vi "tm_setparameterByName.vi"(8 "error in (no error)":errorcluster, 9 "Value":dbl, 10 "Parameter Name":string, 11 "Handle in":u32) -> (0 "error out":errorcluster, 1 "Value out":dbl, 3 "Handle out":u32)   [LabVIEW 2021, in "Camera.lvlib" / "Camera.lvclass"]
uses:
  Camera.lvclass
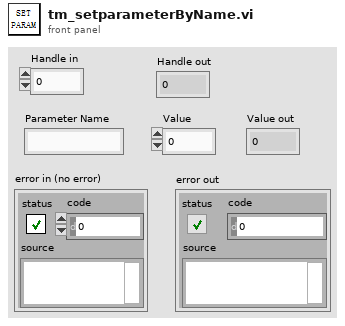
[diagram p1: front panel]
types:
  T1 = cluster{"Function Name":string, "Function ID":u32}[]
  T2 = cluster{"Range":cluster{"min":dbl, "max":dbl, "step":dbl}, "default":dbl, "views":u32, "Writable":bool, "Text Values":bool, "Value Names":cluster{"Name":string, "Value":dbl}[]}
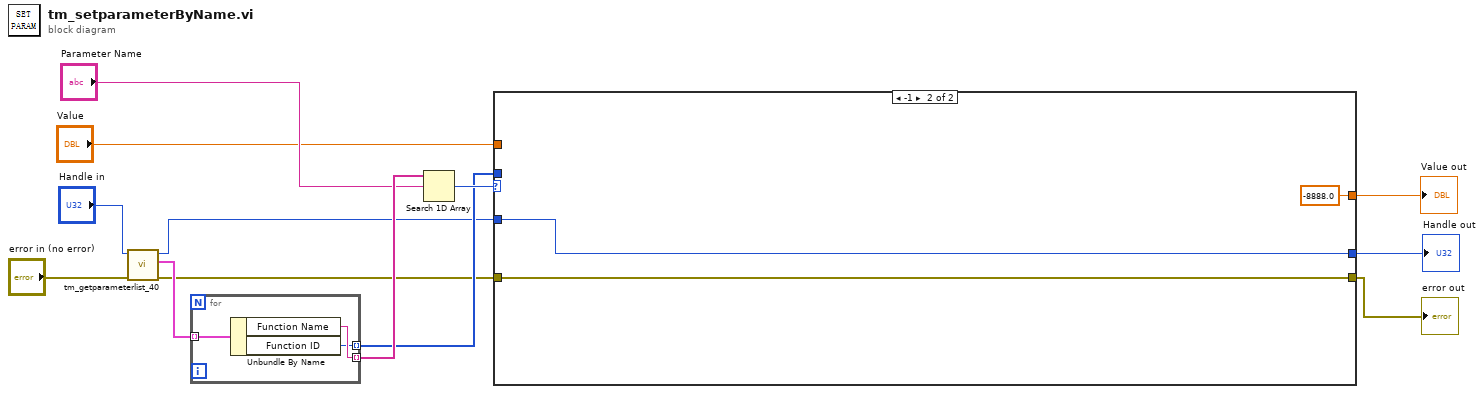
[diagram p0: block diagram]
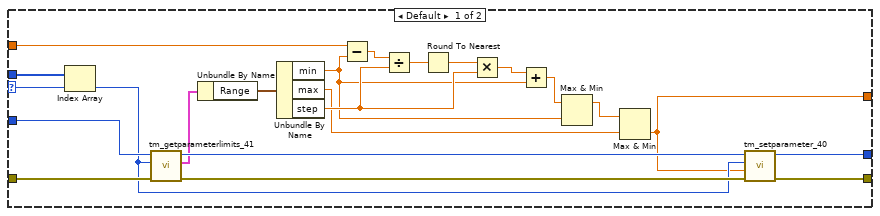
[diagram p2: hidden frame]
diagram:
  n1 = call <userlib>:"tm_getparameterlist_40.vi"("error in (no error)"="error in (no error)", "Handle in"="Handle in") -> ("error out"=w5:errorcluster, "Function List"=w11:T1, "Handle out"=w6:u32)  [unwired: 7 in]
  n2 = for {
    tunnel: w11 -> [w16] mode=indexing
    tunnel: [w15] -> w10 mode=indexing
    tunnel: [w14] -> w7 mode=indexing
    n3 = Unbundle By Name(w16) -> ("Function Name"=w15:string, "Function ID"=w14:u32)
  }
  n4 = Search 1D Array(1D array=w10, element="Parameter Name") -> (index of element=w8:i32)  [unwired: 1 in]
  n5 = case shown="-1" w8 {
    selector: w8 -> [w37 _]
    tunnel: w7 -> [w38 _]
    tunnel: w6 -> [w34 w41]
    tunnel: w5 -> [w32 w40]
    tunnel: "Value" -> [w27 _]
    tunnel: [w36 w41] -> w3
    tunnel: [w35 w40] -> w2
    tunnel: [w17 -8888.0] -> w1
    frame Default {
      n6 = Index Array(array=w38, index=w37) -> (element=w29:u32)
      n7 = call <userlib>:"tm_getparameterlimits_41.vi"("error in (no error)"=w32, "Parameter"=w29, "Handle in"=w34) -> ("error out"=w30:errorcluster, "Limits"=w31:T2, "Handle out"=w33:u32)  [unwired: 6 in]
      n8 = Unbundle By Name(w31) -> ("Range"=w28:cluster{"min":dbl, "max":dbl, "step":dbl})
      n9 = Unbundle By Name(w28) -> ("min"=w20:dbl, "max"=w18:dbl, "step"=w23:dbl)
      n10 = Subtract(x=w27, y=w20) -> (x-y=w26:dbl)
      n11 = Divide(x=w26, y=w23) -> (x/y=w25:dbl)
      n12 = Round To Nearest(number=w25) -> (nearest integer value=w24:dbl)
      n13 = Multiply(x=w24, y=w23) -> (x*y=w22:dbl)
      n14 = Add(x=w22, y=w20) -> (x+y=w21:dbl)
      n15 = Max & Min(x=w21, y=w20) -> (max(x,y)=w19:dbl)  [unwired: 1 out]
      n16 = Max & Min(x=w19, y=w18) -> (min(x,y)=w17:dbl)  [unwired: 1 out]
      n17 = call <userlib>:"tm_setparameter_40.vi"("error in (no error)"=w30, "Value in"=w17, "Parameter"=w29, "Handle in"=w33) -> ("error out"=w35:errorcluster, "Handle out"=w36:u32)  [unwired: 6 in]
    }
    frame -1 {
    }
  }
  "Handle out" <- w3
  "error out" <- w2
  "Value out" <- w1
